vi "Drop Message Core.vi"(11 "Launch Job Msg in":refnum<class "Launch Job Msg.lvclass">) -> ()   [LabVIEW 2014, in "CI Mediator.lvlib" / "Launch Job Msg.lvclass"]
doc: "(<B>Filename</B>: Actor Framework.lvlib:Message.lvclass:Drop Message Core.vi)\n\nDefines what a message does if it is in the message queue when the queue is released. At this point, the actor has shut down, so it will never process the message.\n\nBy default, this method does nothing. A child class may override it to define behavior. National Instruments provides the Reply Msg class to override this method. This class releases its internal queue, which causes any caller of the Send Message and Wait For Response method to stop waiting and return an error."
uses:
  Launch Job Msg.lvclass
  Launch Job Msg.lvclass/Launch Job Msg.ctl
  Controls/Job Results - STYP.ctl
  <vilib>/ActorFramework/Message/Message.lvclass
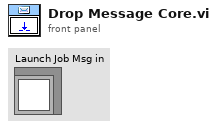
[diagram p1: front panel]
types:
  T1 = typedef "Job Results - STYP.ctl" = cluster{"Status":u16, "Text":string, "Executor Number":i32}
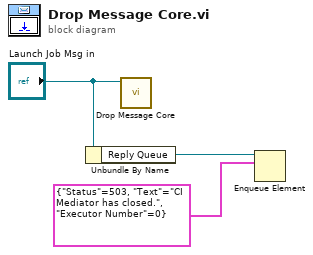
[diagram p0: block diagram]
diagram:
  n1 = Unbundle By Name("Launch Job Msg in") -> ("Reply Queue"=w2:refnum<queue>)
  n2 = call-parent "Drop Message Core.vi"("Message in"="Launch Job Msg in") -> ()  [unwired: 11 in]
  n3 = Enqueue Element(queue=w2, element=T1 {"Status"=503, "Text"="CI Mediator has closed.", "Executor Number"=0}) -> ()  [unwired: 2 in, 3 out]
